vi "Chnl_2_tab.vi"(7 "Command":T3, 8 "Error In":errorcluster, 10 "Tab IN":T2, 11 "Channel IN":T1) -> (0 "Error Out":errorcluster, 2 "Tab Out":T2, 3 "Channel  OUT":T1)   [LabVIEW 2012]
uses:
  Chnl_2_tab_Commands.ctl
  Custom Controls/MAIN Image panel tab Control type def.ctl
  Custom Control and Typedefs/ChannelSelector_for_PosSave.ctl
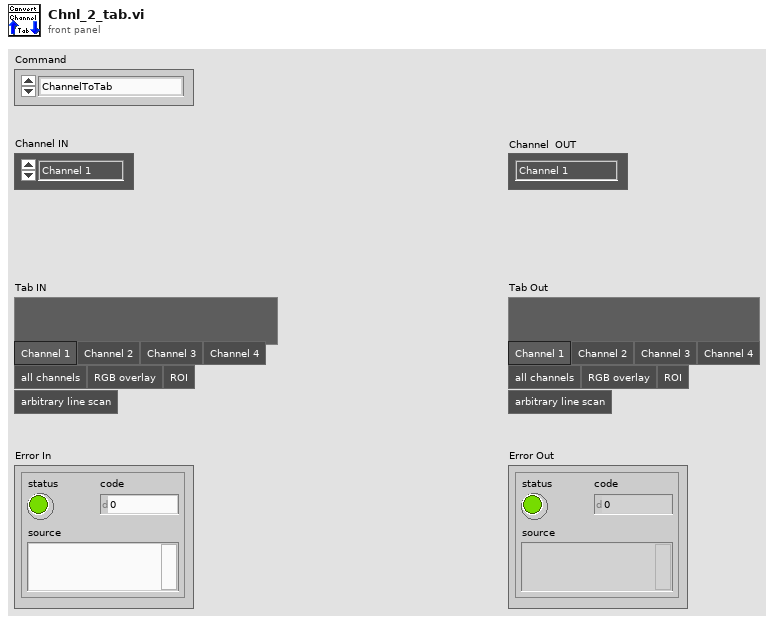
[diagram p1: front panel]
types:
  T1 = typedef "ChannelSelector_for_PosSave.ctl" = enum16{"Channel 1", "Channel 2", "Channel 3", "Channel 4"}
  T2 = typedef "MAIN Image panel tab Control type def.ctl" = enum32{"Channel 1", "Channel 2", "Channel 3", "Channel 4", "all channels", "RGB overlay", "ROI", "arbitrary line scan"}
  T3 = typedef "Chnl_2_tab_Commands.ctl" = enum16{"ChannelToTab", "TabToChannel"}
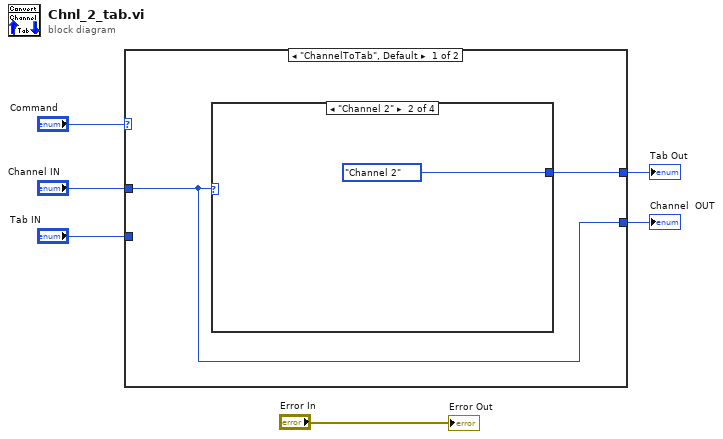
[diagram p0: block diagram]
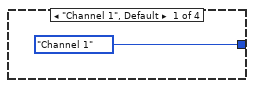
[diagram p2: hidden frame]
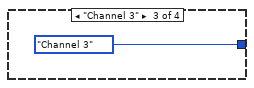
[diagram p3: hidden frame]
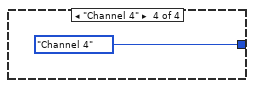
[diagram p4: hidden frame]
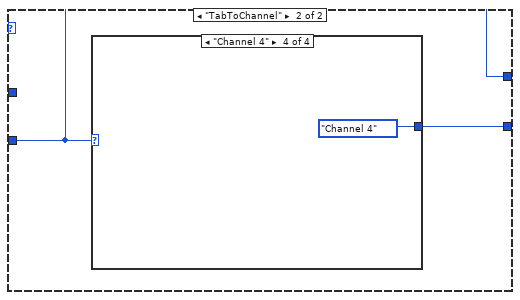
[diagram p5: hidden frame]
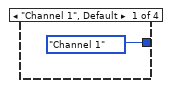
[diagram p6: hidden frame]
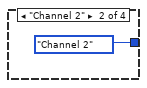
[diagram p7: hidden frame]
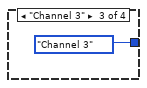
[diagram p8: hidden frame]
diagram:
  n1 = case shown="\"ChannelToTab\", Default" "Command" {
    tunnel: "Channel IN" -> [w7 _]
    tunnel: [w8 w13] -> w4
    tunnel: "Tab IN" -> [_ w13]
    tunnel: [w7 w14] -> w1
    frame "ChannelToTab", Default {
      n2 = case shown="\"Channel 2\"" w7 {
        tunnel: [MAIN_Image_panel_tab_Control_type_def."Channel 1" ("GUI Tab Out") MAIN_Image_panel_tab_Control_type_def."Channel 2" ("GUI Tab Out") MAIN_Image_panel_tab_Control_type_def."Channel 3" ("GUI Tab Out") MAIN_Image_panel_tab_Control_type_def."Channel 4" ("GUI Tab Out")] -> w8
        frame "Channel 1", Default {
        }
        frame "Channel 2" {
        }
        frame "Channel 3" {
        }
        frame "Channel 4" {
        }
      }
    }
    frame "TabToChannel" {
      n3 = case shown="\"Channel 4\"" w13 {
        tunnel: [ChannelSelector_for_PosSave."Channel 1" ("Channel  OUT") ChannelSelector_for_PosSave."Channel 2" ("Channel  OUT") ChannelSelector_for_PosSave."Channel 3" ("Channel  OUT") ChannelSelector_for_PosSave."Channel 4" ("Channel  OUT")] -> w14
        frame "Channel 1", Default {
        }
        frame "Channel 2" {
        }
        frame "Channel 3" {
        }
        frame "Channel 4" {
        }
      }
    }
  }
  "Tab Out" <- w4
  "Channel  OUT" <- w1
  "Error Out" <- "Error In"
